vi "SetParam.vi"(8 "error in (no error)":errorcluster caption="entrée d'erreur (pas d'erreur)", 10 "RepeatedKFold":T1={"n_splits"=5, "n_repeats"=10, "random_state"=-1} {"random_state" min=-1}, 11 "RepeatedKFold.lvclass":refnum<class "RepeatedKFold.lvclass">) -> (0 "error out":errorcluster caption="sortie d'erreur", 3 "RepeatedKFold.lvclass":refnum<class "RepeatedKFold.lvclass">)   [LabVIEW 2020, in "RepeatedKFold.lvclass"]
doc: "Set Parameters"
uses:
  RepeatedKFold.lvclass
  RepeatedKFold.lvclass/RepeatedKFold.ctl
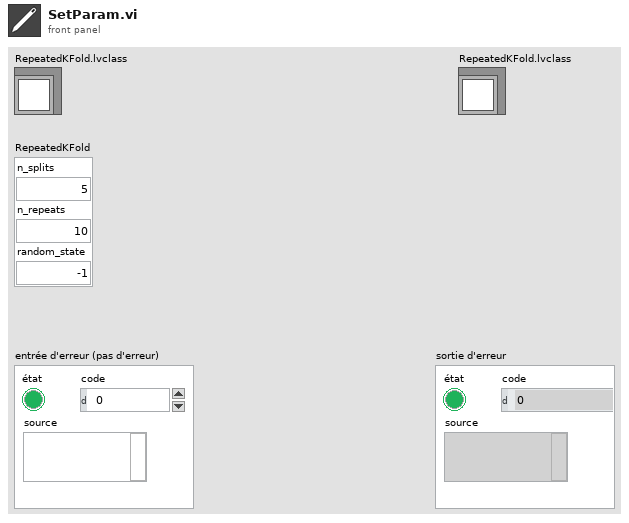
[diagram p1: front panel]
types:
  T1 = cluster{"n_splits":i32, "n_repeats":i32, "random_state":i32}
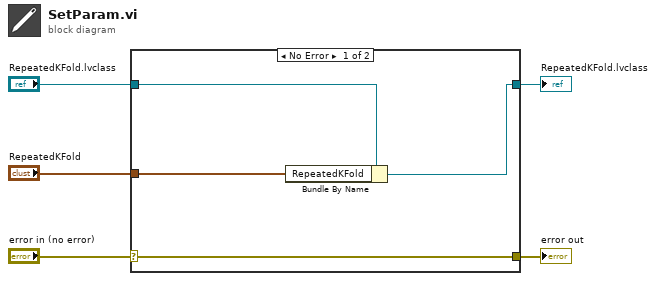
[diagram p0: block diagram]
diagram:
  n1 = case shown="No Error" "error in (no error)" {
    selector: "error in (no error)" -> [w9 w10]
    tunnel: [w9 w10] -> w4
    tunnel: [w7 w11] -> w2
    tunnel: "RepeatedKFold.lvclass" -> [w8 w11]
    tunnel: "RepeatedKFold" -> [w6 _]
    frame No Error {
      n2 = Bundle By Name(cluster=w8, "RepeatedKFold"=w6) -> (w7:refnum<class "RepeatedKFold.lvclass">)
    }
    frame Error {
    }
  }
  "error out" <- w4
  "RepeatedKFold.lvclass" <- w2
